vi "gpanel_DO_move_xy.vi"(8 "error in (no error)":errorcluster, 9 "Y Position":dbl, 10 "X Position":dbl, 11 "galvo_panel in":refnum<class "galvo_panel.lvclass">) -> (0 "error out":errorcluster, 3 "galvo_panel out":refnum<class "galvo_panel.lvclass">)   [LabVIEW 2015, in "galvo_panel.lvclass"]
uses:
  galvo_panel.lvclass
  galvo/galvo.lvclass
  UI/panel_class/panel.lvclass
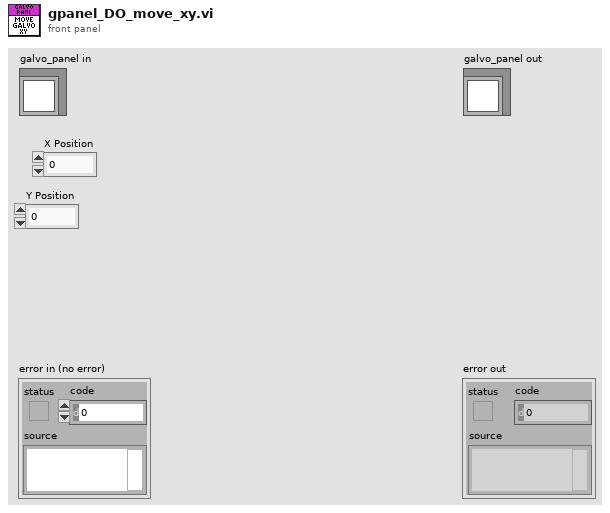
[diagram p1: front panel]
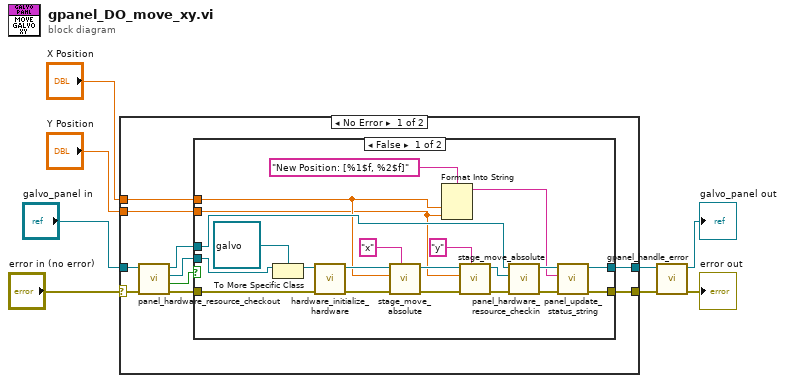
[diagram p0: block diagram]
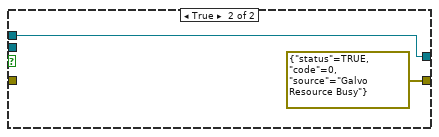
[diagram p2: hidden frame]
diagram:
  n1 = case shown="No Error" "error in (no error)" {
    selector: "error in (no error)" -> [w17 w43]
    tunnel: [w14 w43] -> w4
    tunnel: [w9 w42] -> w2
    tunnel: "galvo_panel in" -> [w18 w42]
    tunnel: "X Position" -> [w12 _]
    tunnel: "Y Position" -> [w11 _]
    frame No Error {
      n2 = call "panel_hardware_resource_checkout.vi"("error in (no error)"=w17, "panel in"=w18) -> ("error out"=w15:errorcluster, "timed out?"=w16:bool, "hardware.lvclass"=w13:refnum<class "hardware.lvclass">, "panel out"=w10:refnum<class "galvo_panel.lvclass">)  [unwired: 6 in]
      n3 = case shown="False" w16 {
        tunnel: [w24 errorcluster {"status"=TRUE, "code"=0, "source"="Galvo Resource Busy"} ("error out")] -> w14
        tunnel: w15 -> [w28 _]
        tunnel: w13 -> [w39 _]
        tunnel: w12 -> [w21 _]
        tunnel: w11 -> [w20 _]
        tunnel: w10 -> [w31 w40]
        tunnel: [w23 w40] -> w9
        frame False {
          n4 = To More Specific Class(target class=refnum<class "galvo.lvclass"> refnum ("galvo.lvclass"), reference=w39) -> (specific class reference=w30:refnum<class "galvo.lvclass">)  [unwired: 1 in, 1 out]
          n5 = call-dynamic "hardware_initialize_hardware.vi"("error in (no error)"=w28, "galvo in"=w30) -> ("error out"=w27:errorcluster, "galvo out"=w29:refnum<class "galvo.lvclass">)  [unwired: 8 in]
          n6 = call-dynamic "stage_move_absolute.vi"("Stage Name"="x", "error in (no error)"=w27, "Position"=w21, "galvo in"=w29) -> ("error out"=w35:errorcluster, "galvo out"=w36:refnum<class "galvo.lvclass">)  [unwired: 6 in]
          n7 = Format Into String(format string="New Position: [%1$f, %2$f]", w21, w20) -> (resulting string=w22:string)  [unwired: 2 in, 1 out]
          n8 = call-dynamic "stage_move_absolute.vi"("Stage Name"="y", "error in (no error)"=w35, "Position"=w20, "galvo in"=w36) -> ("error out"=w33:errorcluster, "galvo out"=w32:refnum<class "galvo.lvclass">)  [unwired: 6 in]
          n9 = call "panel_hardware_resource_checkin.vi"("error in (no error)"=w33, "hardware.lvclass"=w32, "panel in"=w31) -> ("error out"=w25:errorcluster, "panel out"=w26:refnum<class "galvo_panel.lvclass">)  [unwired: 7 in]
          n10 = call-dynamic "panel_update_status_string.vi"("error in (no error)"=w25, "String"=w22, "galvo_panel in"=w26) -> ("error out"=w24:errorcluster, "galvo_panel out"=w23:refnum<class "galvo_panel.lvclass">)  [unwired: 7 in]
        }
        frame True {
        }
      }
    }
    frame Error {
    }
  }
  n11 = call "gpanel_handle_error.vi"("error in (no error)"=w4, "galvo_panel in"=w2) -> ("error out"=→"error out":errorcluster, "galvo_panel out"=→"galvo_panel out":refnum<class "galvo_panel.lvclass">)  [unwired: 8 in]
